vi "Set Ramping Mode.vi"(8 "error in":T2, 9 "Ramping Mode":u16(ring) items=["RAMP", "PAUSE", "MANUAL UP", "MANUAL DOWN", "ZERO"], 11 "Communications Config":T1={"connection ID"=refnum, "IP"="192.168.0.108", "Active Comm Interface"=0, "Serial Port"="", "Programmer Type"=0, "connection ID"=refnum, "output cluster"={"GPIB address"=0, "GPIB bus"=0}} {"Programmer Type" items=["Model 430", "Model 420"]; "Active Comm Interface" items=["TCP/IP (Model 430 Only)", "RS232", "IEEE488"]}) -> (0 "error out":T2)   [LabVIEW 2017]
uses:
  commsControl.ctl
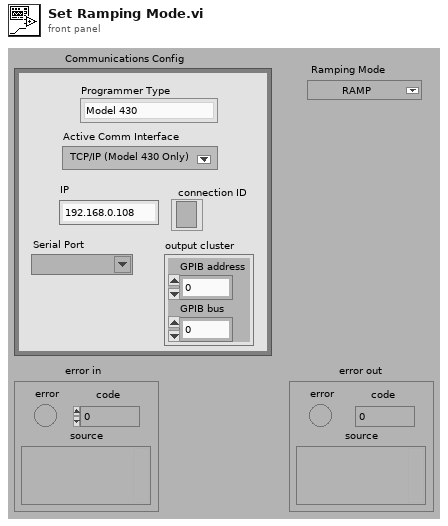
[diagram p1: front panel]
types:
  T1 = typedef "commsControl.ctl" = cluster{"connection ID":refnum<k5>, "IP":string, "Active Comm Interface":u16, "Serial Port":refnum<visa-resource-name>, "Programmer Type":u16, "connection ID":refnum<k5>, "output cluster":cluster{"GPIB address":i16, "GPIB bus":i16}}
  T2 = cluster{"error":bool, "code":i32, "source":string}
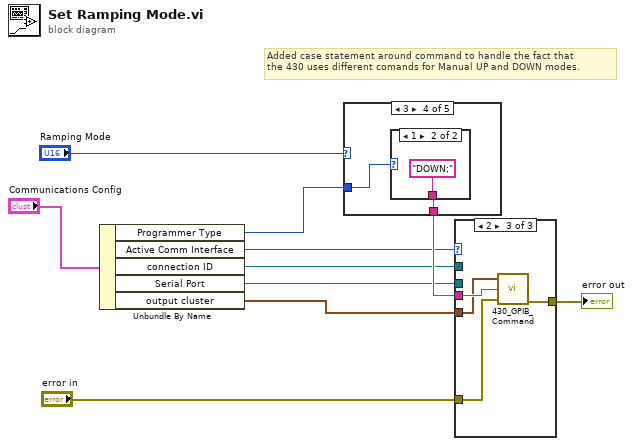
[diagram p0: block diagram]
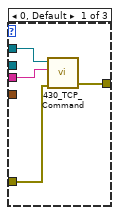
[diagram p2: hidden frame]
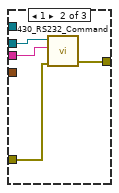
[diagram p3: hidden frame]
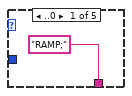
[diagram p4: hidden frame]
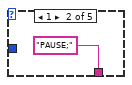
[diagram p5: hidden frame]
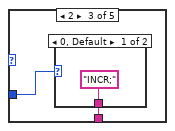
[diagram p6: hidden frame]
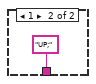
[diagram p7: hidden frame]
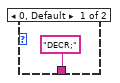
[diagram p8: hidden frame]
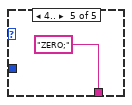
[diagram p9: hidden frame]
diagram:
  # "Added case statement around command to handle the fact that\nthe 430 uses different comands for Manual UP and DOWN modes."
  n1 = Unbundle By Name("Communications Config") -> ("Programmer Type"=w2:u16, "Active Comm Interface"=w3:u16, "connection ID"=w8:refnum<k5>, "Serial Port"=w7:refnum<visa-resource-name>, "output cluster"=w1:cluster{"GPIB address":i16, "GPIB bus":i16})
  n2 = case shown="3" "Ramping Mode" {
    tunnel: w2 -> [_ _ w14 w18 _]
    tunnel: ["RAMP;" "PAUSE;" w13 w17 "ZERO;"] -> w9
    frame ..0 {
    }
    frame 1 {
    }
    frame 2 {
      n3 = case shown="0, Default" w14 {
        tunnel: ["INCR;" "UP;"] -> w13
        frame 0, Default {
        }
        frame 1 {
        }
      }
    }
    frame 3 {
      n4 = case shown="1" w18 {
        tunnel: ["DECR;" "DOWN;"] -> w17
        frame 0, Default {
        }
        frame 1 {
        }
      }
    }
    frame 4.. {
    }
  }
  n5 = case shown="2" w3 {
    tunnel: w7 -> [_ w26 _]
    tunnel: "error in" -> [w24 w28 w33]
    tunnel: w9 -> [w23 w27 w32]
    tunnel: [w25 w29 w31] -> w5
    tunnel: w8 -> [w22 _ _]
    tunnel: w1 -> [_ _ w30]
    frame 0, Default {
      n6 = call "430_TCP_Command.vi"("error in (no error)"=w24, "Command"=w23, "connection ID"=w22) -> ("error out"=w25:errorcluster)  [unwired: 1 in, 2 out]
    }
    frame 1 {
      n7 = call "430_RS232_Command.vi"("error in (no error)"=w28, "Command"=w27, "VISA resource name"=w26) -> ("error out"=w29:errorcluster)  [unwired: 1 in, 2 out]
    }
    frame 2 {
      n8 = call "430_GPIB_Command.vi"("GPIB (In)"=w30, "Input command"=w32, "error in"=w33) -> ("error out"=w31:T2)  [unwired: 3 out]
    }
  }
  "error out" <- w5
